vi "Pfeiffer_Convert_to_Eng.vi"(7 "W/R [W: Int in; Str out ]":bool, 8 "Kommastellen":u8=2, 9 "Eng2 in":dbl format="%.2e", 10 "Eng1 in":dbl format="%.2e", 11 "String in":string) -> (1 "Eng2 out":dbl format="%.2e", 2 "Eng1 out":dbl format="%.2e", 3 "String out":string)   [LabVIEW 2010]
doc: "VI runs with Single / Dual Gauge (TPG 252 / 261 / 262)"
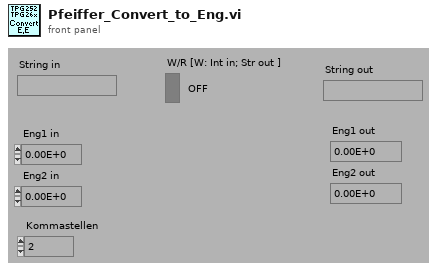
[diagram p1: front panel]
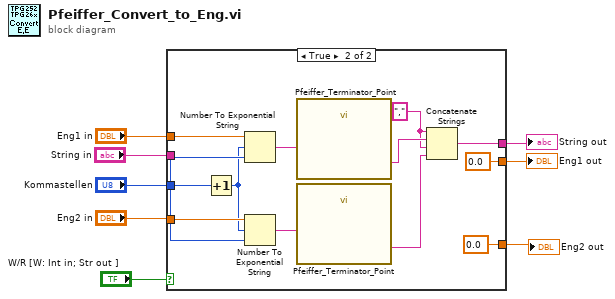
[diagram p0: block diagram]
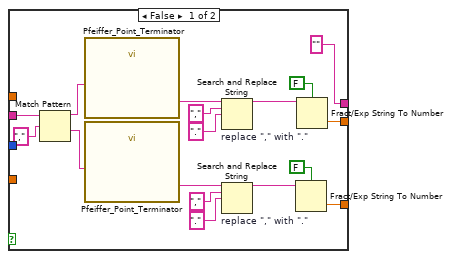
[diagram p2: hidden frame]
diagram:
  n1 = case shown="True" "W/R [W: Int in; Str out ]" {
    tunnel: "Eng1 in" -> [_ w37]
    tunnel: "Eng2 in" -> [_ w36]
    tunnel: ["" w31] -> w5
    tunnel: "String in" -> [w24 _]
    tunnel: [w23 0.0] -> w3
    tunnel: [w22 0.0] -> w2
    tunnel: "Kommastellen" -> [_ w27]
    frame False {
      n2 = Match Pattern(string=w24, regular expression=",") -> (before substring=w15:string, after substring=w20:string)  [unwired: 3 out]
      n3 = call "Pfeiffer_Point_Terminator.vi"("Eingangstring"=w15) -> ("Ausgangstring"=w17:string)
      n4 = call "Pfeiffer_Point_Terminator.vi"("Eingangstring"=w20) -> ("Ausgangstring"=w12:string)
      n5 = Search and Replace String "replace \",\" with \".\""(input string=w17, search string="," ("substring (\"\")"), replace string="." ("substring (\"\")")) -> (result string=w16:string)  [unwired: 1 in, 7 out]
      n6 = Search and Replace String "replace \",\" with \".\""(input string=w12, search string="," ("substring (\"\")"), replace string="." ("substring (\"\")")) -> (result string=w11:string)  [unwired: 1 in, 7 out]
      n7 = Fract/Exp String To Number(use system decimal point (T)=FALSE, string=w11) -> (number=w23:dbl)  [unwired: 3 out]
      n8 = Fract/Exp String To Number(use system decimal point (T)=FALSE, string=w16) -> (number=w22:dbl)  [unwired: 3 out]
    }
    frame True {
      w28 = ","
      n9 = Increment(x=w27) -> (x+1=w26:u8)
      n10 = Number To Exponential String(number=w37, precision (6)=w27, 3:w26) -> (E-format string=w35:string)  [unwired: 1 out]
      n11 = Number To Exponential String(number=w36, precision (6)=w27, 3:w26) -> (E-format string=w34:string)  [unwired: 1 out]
      n12 = call "Pfeiffer_Terminator_Point.vi"("Eingangstring"=w35) -> ("Ausgangstring"=w33:string)
      n13 = call "Pfeiffer_Terminator_Point.vi"("Eingangstring"=w34) -> ("Ausgangstring"=w32:string)
      n14 = Concatenate Strings(w28, w33, w28, w32) -> (w31:string)
    }
  }
  "String out" <- w5
  "Eng1 out" <- w2
  "Eng2 out" <- w3
